vi "PSVCH_Run.vi"(8 "Error In (no error)":errorcluster, 11 "Q_EG Name":string) -> (0 "Error Out":errorcluster)   [LabVIEW 2016]
panel:
  # "Data Out"
  # "Data In"
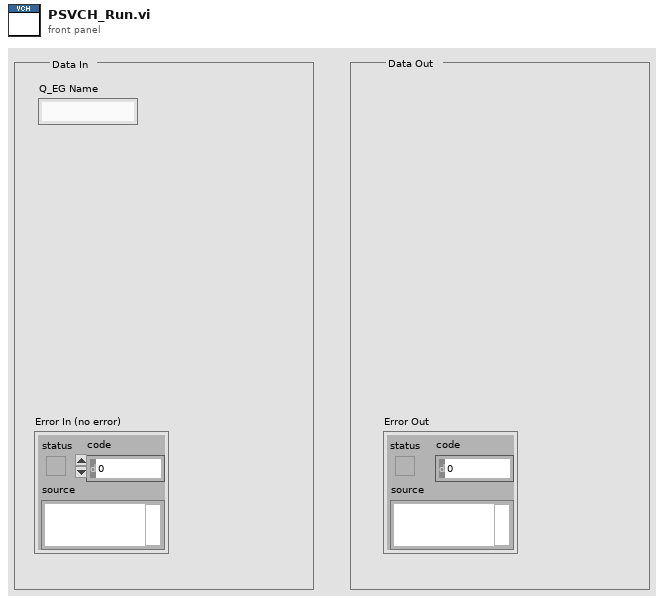
[diagram p1: front panel]
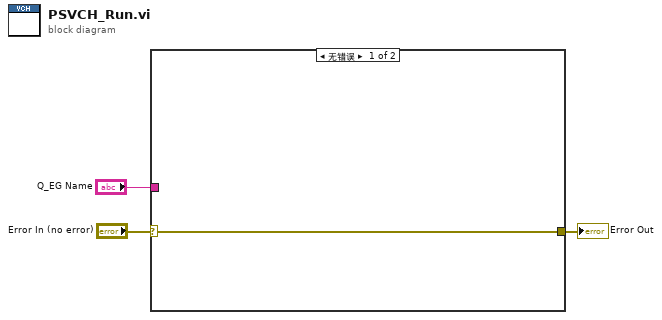
[diagram p0: block diagram]
diagram:
  n1 = case shown="无错误" "Error In (no error)" {
    selector: "Error In (no error)" -> [w4 w5]
    tunnel: [w4 w5] -> w2
    tunnel: "Q_EG Name" -> [_ _]
    frame No Error {
    }
    frame Error {
    }
  }
  "Error Out" <- w2
